vi "Load_Template_Globals.vi"(1 "Channel Names":string[](array[string]), 2 "Template-read":path) -> (0 "Valid Template File?":bool)   [LabVIEW 2016]
uses:
  Data plotting/subVIs/Dispose_Channel.ctl
  Controls/Global_mode.ctl
  Results_plotter_Global.vi
panel:
  in  "Dispose":T1
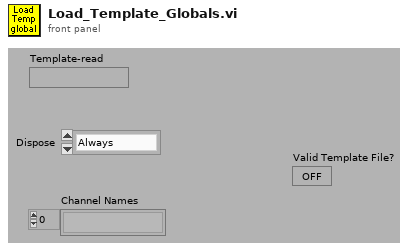
[diagram p1: front panel]
types:
  T1 = typedef "Dispose_Channel.ctl" = enum16{"Always", "If Blank", "Never"}
  T2 = typedef "Global_mode.ctl" = enum16{"Read Global", "Load Global From File", "Write Global to File"}
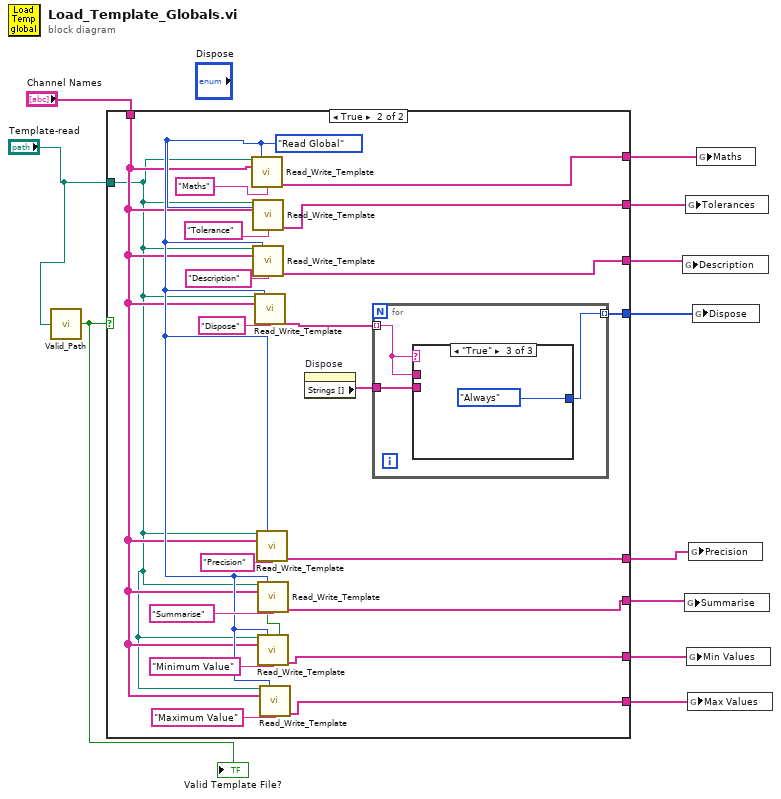
[diagram p0: block diagram]
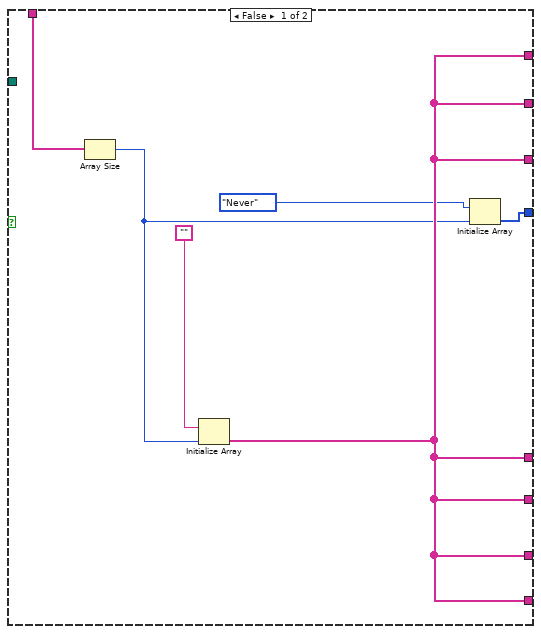
[diagram p2: hidden frame]
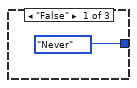
[diagram p3: hidden frame]
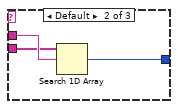
[diagram p4: hidden frame]
diagram:
  n1 = call "Valid_Path.vi"("Filename"="Template-read") -> ("Valid Path?"=w4:bool)
  "Valid Template File?" <- w4
  n2 = case shown="True" w4 {
    tunnel: "Template-read" -> [_ w23]
    tunnel: "Channel Names" -> [w16 w24]
    tunnel: [w15 w34] -> w7
    tunnel: [w15 w33] -> w8
    tunnel: [w14 w19] -> w9
    tunnel: [w15 w32] -> w10
    tunnel: [w15 w31] -> w11
    tunnel: [w15 w29] -> w3
    tunnel: [w15 w22] -> w2
    tunnel: [w15 w21] -> w1
    frame False {
      n3 = Array Size(array=w16) -> (size(s)=w13:i32)
      n4 = Initialize Array("", w13) -> (w15:string[])
      n5 = Initialize Array(Dispose_Channel."Never" ("Dispose"), w13) -> (w14:T1[])
    }
    frame True {
      w25 = Global_mode."Read Global" ("Mode")
      n6 = call "Read_Write_Template.vi"("Template File"=w23, "Mode"=w25, "Channel names In"=w24, "Data type"="Maths") -> ("1D Info Out"=w29:string[])  [unwired: 4 in, 7 out]
      n7 = call "Read_Write_Template.vi"("Template File"=w23, "Mode"=w25, "Channel names In"=w24, "Data type"="Tolerance") -> ("1D Info Out"=w31:string[])  [unwired: 4 in, 7 out]
      n8 = call "Read_Write_Template.vi"("Template File"=w23, "Mode"=w25, "Channel names In"=w24, "Data type"="Description") -> ("1D Info Out"=w32:string[])  [unwired: 4 in, 7 out]
      n9 = call "Read_Write_Template.vi"("Template File"=w23, "Mode"=w25, "Channel names In"=w24, "Data type"="Dispose") -> ("1D Info Out"=w20:string[])  [unwired: 4 in, 7 out]
      n10 = call "Read_Write_Template.vi"("Template File"=w23, "Mode"=w25, "Channel names In"=w24, "Data type"="Precision") -> ("1D Info Out"=w33:string[])  [unwired: 4 in, 7 out]
      n11 = call "Read_Write_Template.vi"("Template File"=w23, "Mode"=w25, "Channel names In"=w24, "Data type"="Minimum Value") -> ("Freshly Loaded?"=w27:bool, "1D Info Out"=w22:string[])  [unwired: 4 in, 6 out]
      n12 = call "Read_Write_Template.vi"("Template File"=w23, "Mode"=w25, "Channel names In"=w24, "Save file"=w27, "Data type"="Summarise") -> ("1D Info Out"=w34:string[])  [unwired: 3 in, 7 out]
      n13 = call "Read_Write_Template.vi"("Template File"=w23, "Mode"=w25, "Channel names In"=w24, "Data type"="Maximum Value") -> ("1D Info Out"=w21:string[])  [unwired: 4 in, 7 out]
      n14 = property on="Dispose" class="Enum (strict)"() -> ("Strings []"=w18:string[])  [unwired: 2 in, 2 out]
      n15 = for {
        tunnel: w20 -> [w42] mode=indexing
        tunnel: [w40] -> w19 mode=indexing
        tunnel: w18 -> [w41]
        n16 = case shown="\"True\"" w42 {
          tunnel: w42 -> [_ w46 _]
          tunnel: w41 -> [_ w45 _]
          tunnel: [Dispose_Channel."Never" ("Dispose") w44 Dispose_Channel."Always" ("Dispose")] -> w40
          frame "False" {
          }
          frame Default {
            n17 = Search 1D Array(1D array=w45, element=w46) -> (index of element=w44:i32)  [unwired: 1 in]
          }
          frame "True" {
          }
        }
      }
    }
  }
  n18 = global write "Results_plotter_Global.vi" "Description"(w10) -> ()
  n19 = global write "Results_plotter_Global.vi" "Summarise"(w7) -> ()
  n20 = global write "Results_plotter_Global.vi" "Tolerances"(w11) -> ()
  n21 = global write "Results_plotter_Global.vi" "Min Values"(w2) -> ()
  n22 = global write "Results_plotter_Global.vi" "Max Values"(w1) -> ()
  n23 = global write "Results_plotter_Global.vi" "Precision"(w8) -> ()
  n24 = global write "Results_plotter_Global.vi" "Dispose"(w9) -> ()
  n25 = global write "Results_plotter_Global.vi" "Maths"(w3) -> ()
